vi "ODMR Velmex sweep ACCES DAC control.vi"() -> ()   [LabVIEW 2012]
uses:
  <vilib>/DAQmx/read.llb/DAQmx Read (Counter 1D DBL 1Chan NSamp).vi
  <vilib>/Analysis/1siggen.llb/Ramp Pattern by Samples.vi
  VELMEX step motor/GMW Motion Control_VELMEX_V2_2.llb/Config.vi
  <vilib>/DAQmx/create/channels.llb/DAQmx Create Channel (CI-Count Edges).vi
  <vilib>/DAQmx/configure/timing.llb/DAQmx Timing (Sample Clock).vi
  <vilib>/Utility/file.llb/Write To Spreadsheet File (DBL).vi
  <vilib>/DAQmx/miscellaneous.llb/DAQmx Fill In Error Info.vi
  <resource>/objmgr/daqmx.rc
  <vilib>/Analysis/NI_AALBase.lvlib
panel:
  in  "Home?":bool
  in  "Home T":dbl=50.0
  in  "Home Z":dbl=50.0
  in  "Home Y":dbl=50.0
  in  "Home X":dbl=50.0
  in  "angle":dbl
  in  "angled?":bool
  out "position":dbl
  in  "start":dbl format="%0.2f"
  in  "end":dbl=1.0 format="%0.2f"
  in  "samples":i32=128
  in  "axis":string="T"
  in  "GPIB Address":refnum<visa-resource-name>="GPIB0::1::INSTR"
  in  "datalog path (use dialog)":path
  out "XY Graph":cluster{"Y":dbl[], "Y":dbl[]}[](graph)
  in  "file path (dialog if empty)":path=path "C:/Users/Ouyang Group/Documents/Data/5-13-15/ND Au 686 ODMR sweep 1"
  in  "Z Pos":dbl=52.78
  in  "Y Pos":dbl=112.0
  in  "X Pos":dbl=97.0
  in  "Y Parameters":T1={"Number of Y Steps"=200, "Max Y (V)"=2.0, "Min Y (V)"=-2.0}
  in  "X Parameters":T2={"Number of X Steps"=200, "Max X (V)"=2.0, "Min X (V)"=-2.0}
  in  "RS232 settings":cluster{"Portnumber":i32, "Baudrate":u16}={"Portnumber"=6, "Baudrate"=5} {"Portnumber" items=["COM1", "COM2", "COM3", "COM4", "COM5", "COM6", "COM7", "COM8", "COM9", "COM10", "COM11", "COM12", "COM13", "COM14", "COM15", "COM16", "COM17", "COM18", "COM19", "COM20", "COM21", "COM22", "COM23", "COM24", "COM25", "COM26", "COM27", "COM28", "COM29", "COM30"]; "Baudrate" items=["9600", "14400", "19200", "38400", "57600", "115200"]}
  in  "samples per channel":i32=500
  in  "rate":dbl=100.0 format="%0.2f"
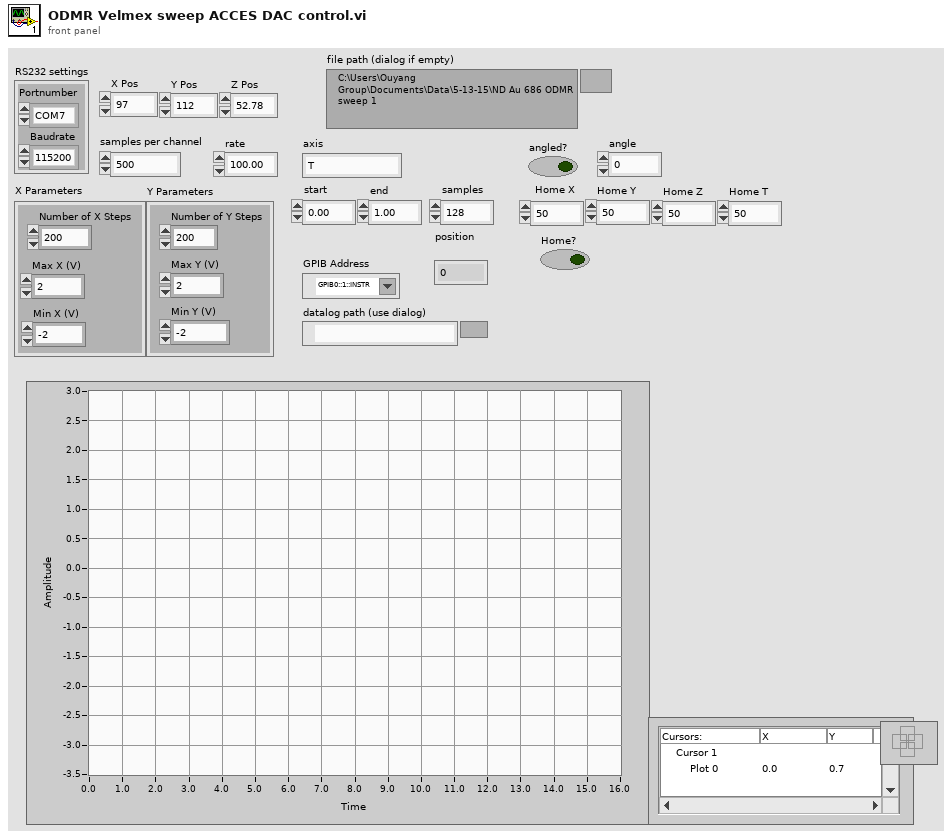
[diagram p1: front panel]
types:
  T1 = cluster{"Number of Y Steps":i32, "Max Y (V)":dbl, "Min Y (V)":dbl}
  T2 = cluster{"Number of X Steps":i32, "Max X (V)":dbl, "Min X (V)":dbl}
  T3 = cluster{"Controller Setup":cluster{"T":string, "Z":string, "Y":string, "X":string, "CW Offset":dbl, "CCW Offset":dbl, "Z Offset":dbl, "Y Offset":dbl, "X Offset":dbl, "Rotary Resolution":i32, "Linear Resolution":i32, "T Speed":dbl, "Z Speed":dbl, "Y Speed":dbl, "X Speed":dbl}, "SoftLimit":cluster{"X soft limit":cluster{"X up soft limit":dbl, "X low soft limit":dbl}, "Y soft limit":cluster{"Y up soft limit":dbl, "Y low soft limit":dbl}, "Z soft limit":cluster{"Z up soft limit":dbl, "Z low soft limit":dbl}, "T soft limit":cluster{"T up soft limit":dbl, "T low soft limit":dbl}}}
  T4 = cluster{"T":string, "Z":string, "Y":string, "X":string, "CW Offset":dbl, "CCW Offset":dbl, "Z Offset":dbl, "Y Offset":dbl, "X Offset":dbl, "Rotary Resolution":i32, "Linear Resolution":i32, "T Speed":dbl, "Z Speed":dbl, "Y Speed":dbl, "X Speed":dbl}
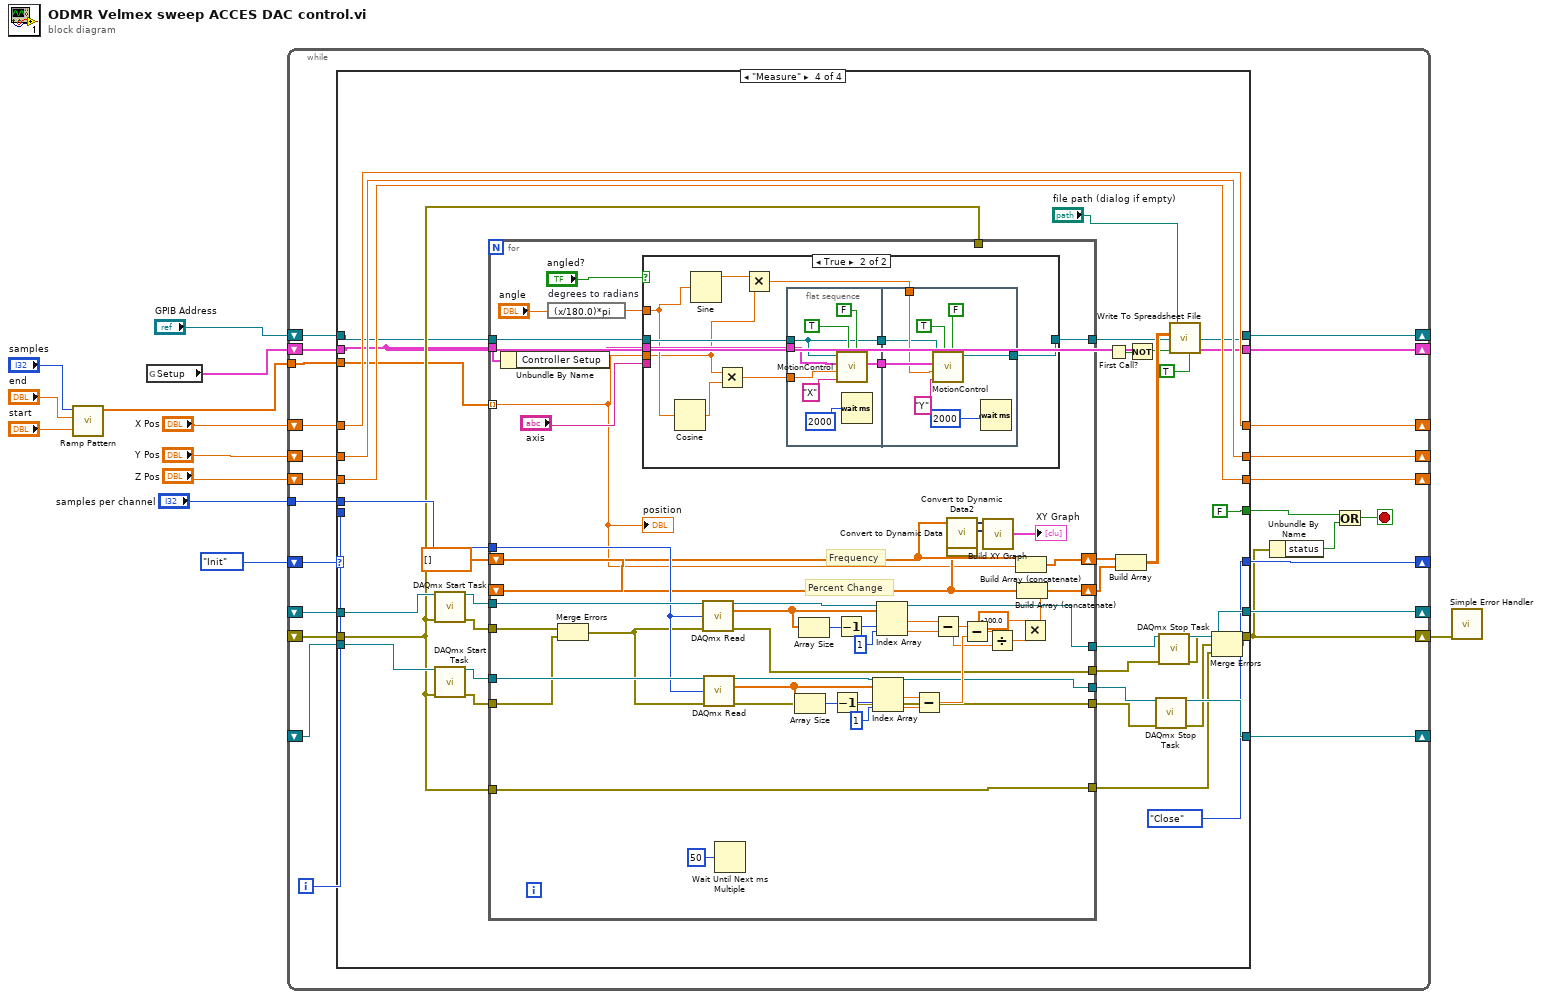
[diagram p0: block diagram]
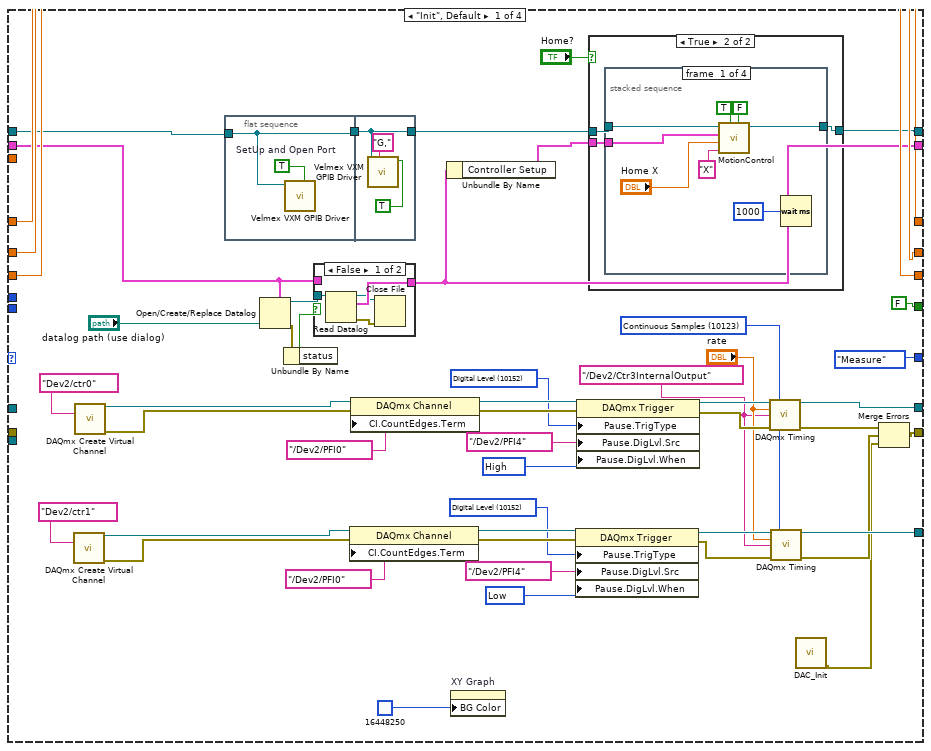
[diagram p2: hidden frame]
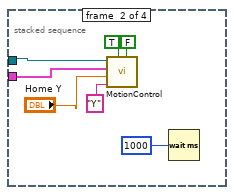
[diagram p4: hidden frame]
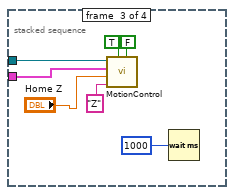
[diagram p5: hidden frame]
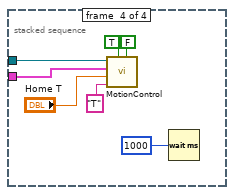
[diagram p6: hidden frame]
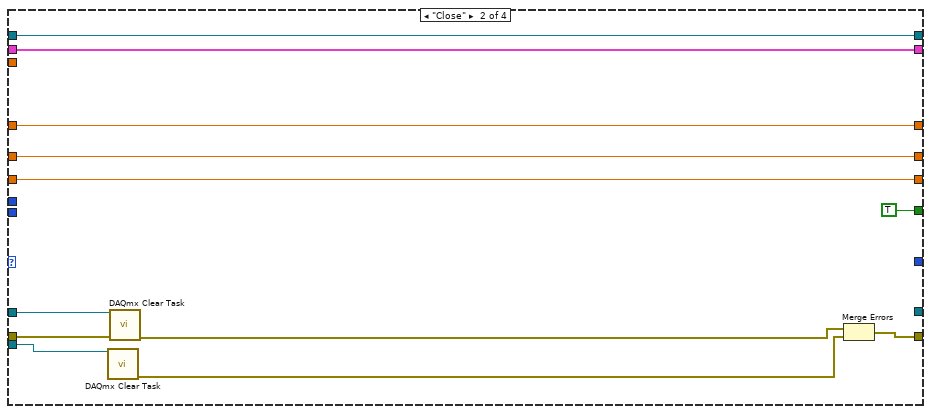
[diagram p8: hidden frame]
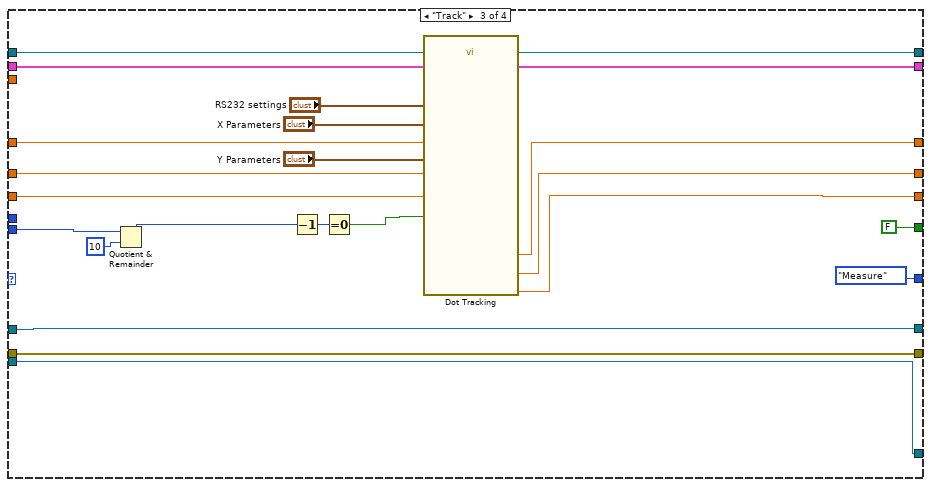
[diagram p9: hidden frame]
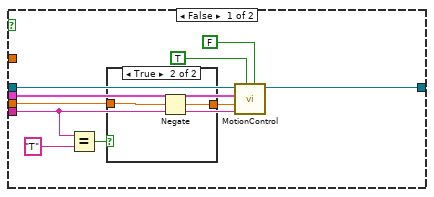
[diagram p10: hidden frame]
diagram:
  n1 = call-poly <vilib>:"Ramp Pattern.vi"("start"="start", "end"="end", "samples"="samples") -> ("Ramp Pattern"=w1:dbl[])  [unwired: 7 in, 1 out]
  n2 = global read "Config.vi" "Setup"() -> (w5:T3)
  n3 = while {
    shift-right: [w33] -> _
    shift-left: enum16{"Init", "Measure", "Track", "Close"}."Init" -> [w36]
    shift-right: [w35] -> _
    shift-left: _ -> [w32]
    shift-right: [w34] -> _
    shift-left: _ -> [w31]
    shift-right: [w28] -> w10
    shift-left: _ -> [w30]
    tunnel: "samples per channel" -> [w25]
    shift-right: [w20] -> _
    shift-left: "X Pos" -> [w23]
    shift-right: [w19] -> _
    shift-left: "Y Pos" -> [w22]
    shift-right: [w18] -> _
    shift-left: "Z Pos" -> [w21]
    shift-right: [w17] -> _
    shift-left: "GPIB Address" -> [w14]
    shift-right: [w16] -> _
    shift-left: w5 -> [w15]
    tunnel: w1 -> [w13]
    i -> [w29]
    stop <- w27 stop-if-true
    n4 = case shown="\"Measure\"" w36 {
      tunnel: [FALSE TRUE FALSE FALSE] -> w26
      tunnel: [w60 _ w161 w186] -> w35
      tunnel: [w59 _ w160 w183] -> w34
      tunnel: [w56 w135 w151 w196] -> w28
      tunnel: [enum16{"Init", "Measure", "Track", "Close"}."Measure" _ enum16{"Init", "Measure", "Track", "Close"}."Measure" enum16{"Init", "Measure", "Track", "Close"}."Close"] -> w33
      tunnel: w32 -> [_ w139 w161 w192]
      tunnel: w31 -> [_ w137 w160 w189]
      tunnel: w30 -> [_ w138 w151 w168]
      tunnel: w29 -> [_ _ w152 _]
      tunnel: w25 -> [_ _ _ w174]
      tunnel: w23 -> [w52 w133 w148 w172]
      tunnel: w22 -> [w51 w132 w147 w171]
      tunnel: w21 -> [w50 w131 w146 w170]
      tunnel: [w52 w133 w145 w172] -> w20
      tunnel: [w51 w132 w144 w171] -> w19
      tunnel: [w50 w131 w143 w170] -> w18
      tunnel: [w40 w130 w142 w163] -> w17
      tunnel: [w39 w129 w141 w164] -> w16
      tunnel: w14 -> [w43 w130 w142 w165]
      tunnel: w15 -> [w42 w129 w141 w164]
      tunnel: w13 -> [_ _ _ w162]
      frame "Init", Default {
        w61 = tag "/Dev2/Ctr3InternalOutput" ("source")
        w63 = 10123 items=["Finite Samples"=10178, "Continuous Samples"=10123, "Hardware Timed Single Point"=12522] ("sample mode")
        w68 = 10214 items=["High"=10192, "Low"=10214] ("Pause.DigLvl.When")
        w70 = 10152 items=["Analog Level"=10101, "Analog Window"=10103, "Digital Level"=10152, "Digital Pattern"=10398, "None"=10230] ("Pause.TrigType")
        w77 = 10192 items=["High"=10192, "Low"=10214] ("Pause.DigLvl.When")
        w79 = 10152 items=["Analog Level"=10101, "Analog Window"=10103, "Digital Level"=10152, "Digital Pattern"=10398, "None"=10230] ("Pause.TrigType")
        n5 = call-poly <vilib>:"DAQmx Create Virtual Channel.vi"("counter"=tag "Dev2/ctr1") -> ("task out"=w75:refnum<k21>, "error out"=w74:errorcluster)  [unwired: 13 in]
        n6 = call-poly <vilib>:"DAQmx Create Virtual Channel.vi"("counter"=tag "Dev2/ctr0") -> ("task out"=w84:refnum<k21>, "error out"=w83:errorcluster)  [unwired: 13 in]
        n7 = flat-sequence {
          tunnel: w43 -> [w119]
          tunnel: [w119] -> w48
          tunnel: [w123] -> w41
          tunnel: w48 -> [w123]
          frame #0 {
            w120 = TRUE  # SetUp and Open Port
            n8 = call "Velmex VXM GPIB Driver.vi"("SetUp and Open Port"=w120, "VISA resource name"=w119) -> ()  [unwired: 8 in, 2 out]
          }
          frame #1 {
            n9 = call "Velmex VXM GPIB Driver.vi"("Send String to VXM"=TRUE, "String to send to VXM"="G,", "VISA resource name"=w123) -> ()  [unwired: 7 in, 2 out]
          }
        }
        n10 = Open/Create/Replace Datalog(5:w42, 11:"datalog path (use dialog)") -> (0:w47:errorcluster, 3:w46:refnum<k1>)  [unwired: 4 in, 1 out]
        n11 = Unbundle By Name(w47) -> ("status"=w45:bool)
        n12 = case shown="False" w45 {
          tunnel: w46 -> [w124 _]
          tunnel: [w127 w128] -> w39
          tunnel: w42 -> [_ w128]
          frame False {
            n13 = Read Datalog(7:w124) -> (0:w126:errorcluster, 2:w127:T3, 3:w125:refnum<k1>)  [unwired: 2 in]
            n14 = Close File(refnum=w125, error in=w126) -> ()  [unwired: 2 out]
          }
          frame True {
          }
        }
        n15 = property class="DAQmx Channel"(reference=w75, error in=w74, "CI.CountEdges.Term"=tag "/Dev2/PFI0") -> (reference out=w72:refnum<k21>, error out=w71:errorcluster)
        n16 = property class="DAQmx Channel"(reference=w84, error in=w83, "CI.CountEdges.Term"=tag "/Dev2/PFI0") -> (reference out=w81:refnum<k21>, error out=w80:errorcluster)
        n17 = Unbundle By Name(w39) -> ("Controller Setup"=w38:T4)
        n18 = property on="XY Graph" class="XYGraph (strict)"("BG Color"=u32 16448250) -> ()  [unwired: 2 in, 2 out]
        n19 = property class="DAQmx Trigger"(reference=w72, error in=w71, "Pause.TrigType"=w70, "Pause.DigLvl.Src"=tag "/Dev2/PFI4", "Pause.DigLvl.When"=w68) -> (reference out=w65:refnum<k21>, error out=w64:errorcluster)
        n20 = property class="DAQmx Trigger"(reference=w81, error in=w80, "Pause.TrigType"=w79, "Pause.DigLvl.Src"=tag "/Dev2/PFI4", "Pause.DigLvl.When"=w77) -> (reference out=w67:refnum<k21>, error out=w66:errorcluster)
        n21 = case shown="True" "Home?" {
          tunnel: w41 -> [w86 w89]
          tunnel: [w86 w88] -> w40
          tunnel: w38 -> [_ w87]
          frame False {
          }
          frame True {
            n22 = stacked-sequence {
              tunnel: [w91 _ _ _] -> w88
              tunnel: w87 -> [w92 w99 w109 w113]
              tunnel: w89 -> [w93 w100 w110 w114]
              frame #0 {
                n23 = call "MotionControl.vi"("STOP motion"=FALSE, "START motion"=TRUE, "axis"="X", "Position"="Home X", "Setup"=w92, "VISA resource name in"=w93) -> ("VISA resource name out"=w91:refnum<visa-resource-name>)  [unwired: 3 in]
                n24 = Wait (ms)(milliseconds to wait=u32 1000) -> ()  [unwired: 1 out]
              }
              frame #1 {
                n25 = call "MotionControl.vi"("STOP motion"=FALSE, "START motion"=TRUE, "axis"="Y", "Position"="Home Y", "Setup"=w99, "VISA resource name in"=w100) -> ()  [unwired: 3 in, 1 out]
                n26 = Wait (ms)(milliseconds to wait=u32 1000) -> ()  [unwired: 1 out]
              }
              frame #2 {
                n27 = call "MotionControl.vi"("STOP motion"=FALSE, "START motion"=TRUE, "axis"="Z", "Position"="Home Z", "Setup"=w109, "VISA resource name in"=w110) -> ()  [unwired: 3 in, 1 out]
                n28 = Wait (ms)(milliseconds to wait=u32 1000) -> ()  [unwired: 1 out]
              }
              frame #3 {
                n29 = call "MotionControl.vi"("STOP motion"=FALSE, "START motion"=TRUE, "axis"="T", "Position"="Home T", "Setup"=w113, "VISA resource name in"=w114) -> ()  [unwired: 3 in, 1 out]
                n30 = Wait (ms)(milliseconds to wait=u32 1000) -> ()  [unwired: 1 out]
              }
            }
          }
        }
        n31 = call-poly <vilib>:"DAQmx Timing.vi"("task/channels in"=w67, "sample mode"=w63, "rate"="rate", "source"=w61, "error in"=w66) -> ("task out"=w60:refnum<k21>, "error out"=w58:errorcluster)  [unwired: 9 in]
        n32 = call-poly <vilib>:"DAQmx Timing.vi"("task/channels in"=w65, "sample mode"=w63, "rate"="rate", "source"=w61, "error in"=w64) -> ("task out"=w59:refnum<k21>, "error out"=w57:errorcluster)  [unwired: 9 in]
        n33 = call "DAC_Init.vi"() -> ("error out"=w49:errorcluster)  [unwired: 11 in]
        n34 = Merge Errors(w58, w57, w49) -> (w56:errorcluster)
      }
      frame "Close" {
        n35 = call <vilib>:"DAQmx Clear Task.vi"("task in"=w137) -> ("error out"=w136:errorcluster)  [unwired: 14 in]
        n36 = call <vilib>:"DAQmx Clear Task.vi"("task in"=w139, "error in"=w138) -> ("error out"=w134:errorcluster)  [unwired: 13 in]
        n37 = Merge Errors(w134, w136) -> (w135:errorcluster)
      }
      frame "Track" {
        n38 = Quotient & Remainder(x=w152, y=10) -> (x-y*floor(x/y)=w155:i32)  [unwired: 1 out]
        n39 = Decrement(x=w155) -> (x-1=w156:i32)
        n40 = Equal To 0?(x=w156) -> (x = 0?=w153:bool)
        n41 = call "Dot Tracking.vi"("X"="X Parameters", "Y Parameters"="Y Parameters", "RS232 settings"="RS232 settings", "X Pos"=w148, "Y pos"=w147, "Z Pos"=w146, "Z-track?"=w153) -> ("X Position"=w145:dbl, "Y Position"=w144:dbl, "Z Position"=w143:dbl)  [unwired: 2 in, 4 out]
      }
      frame "Measure" {
        w173 = dbl[] []
        n42 = call <vilib>:"DAQmx Start Task.vi"("task/channels in"=w192, "error in"=w168) -> ("task out"=w190:refnum<k21>, "error out"=w191:errorcluster)  [unwired: 12 in]
        n43 = call <vilib>:"DAQmx Start Task.vi"("task/channels in"=w189, "error in"=w168) -> ("task out"=w188:refnum<k21>, "error out"=w187:errorcluster)  [unwired: 12 in]
        n44 = for {
          shift-right: [w229] -> w180
          shift-left: w173 -> [w215]
          shift-right: [w228] -> w181
          shift-left: w173 -> [w217]
          tunnel: w188 -> [w224]
          tunnel: [w223] -> w185
          tunnel: [w222] -> w194
          tunnel: [w219] -> w193
          tunnel: w191 -> [w221]
          tunnel: w190 -> [w220]
          tunnel: w187 -> [w210]
          tunnel: w174 -> [w218]
          tunnel: w168 -> [_]
          tunnel: [w208] -> w169
          tunnel: w168 -> [w201]
          tunnel: [w201] -> w167
          tunnel: w165 -> [w206]
          tunnel: w164 -> [w205]
          tunnel: [w202] -> w163
          tunnel: w162 -> [w200] mode=indexing
          # "Percent Change"
          # "Frequency"
          n45 = Unbundle By Name(w205) -> ("Controller Setup"=w203:T4)
          n46 = expression code="(x/180.0)*pi" "degrees to radians"("angle") -> (w197:dbl)
          n47 = Merge Errors(w221, w210) -> (w209:errorcluster)
          n48 = case shown="True" "angled?" {
            tunnel: w206 -> [w250 w266]
            tunnel: "axis" -> [w247 _]
            tunnel: w203 -> [w249 w265]
            tunnel: [w248 w260] -> w202
            tunnel: w200 -> [w244 w258]
            tunnel: w197 -> [_ w264]
            frame False {
              n49 = Equal?(x=w247, y="T") -> (x = y?=w245:bool)
              n50 = case shown="True" w245 {
                tunnel: w244 -> [w253 w255]
                tunnel: [w253 w254] -> w243
                frame False {
                }
                frame True {
                  n51 = Negate(x=w255) -> (-x=w254:dbl)
                }
              }
              n52 = call "MotionControl.vi"("STOP motion"=FALSE, "START motion"=TRUE, "axis"=w247, "Position"=w243, "Setup"=w249, "VISA resource name in"=w250) -> ("VISA resource name out"=w248:refnum<visa-resource-name>)  [unwired: 3 in]
            }
            frame True {
              n53 = Cosine(x=w264) -> (cos(x)=w263:dbl)
              n54 = Sine(x=w264) -> (sin(x)=w259:dbl)
              n55 = Multiply(x=w258, y=w263) -> (x*y=w262:dbl)
              n56 = Multiply(x=w259, y=w258) -> (x*y=w257:dbl)
              n57 = flat-sequence {
                tunnel: w266 -> [w268]
                tunnel: w265 -> [w267]
                tunnel: w262 -> [w270]
                tunnel: [w267] -> w261
                tunnel: [w268] -> w256
                tunnel: w261 -> [w278]
                tunnel: [w277] -> w260
                tunnel: w257 -> [w276]
                tunnel: w256 -> [w275]
                frame #0 {
                  n58 = call "MotionControl.vi"("STOP motion"=FALSE, "START motion"=TRUE, "axis"="X", "Position"=w270, "Setup"=w267, "VISA resource name in"=w268) -> ()  [unwired: 3 in, 1 out]
                  n59 = Wait (ms)(milliseconds to wait=u32 2000 ("millisecond multiple")) -> ()  [unwired: 1 out]
                }
                frame #1 {
                  n60 = call "MotionControl.vi"("STOP motion"=FALSE, "START motion"=TRUE, "axis"="Y", "Position"=w276, "Setup"=w278, "VISA resource name in"=w275) -> ("VISA resource name out"=w277:refnum<visa-resource-name>)  [unwired: 3 in]
                  n61 = Wait (ms)(milliseconds to wait=u32 2000 ("millisecond multiple")) -> ()  [unwired: 1 out]
                }
              }
            }
          }
          n62 = call-poly <vilib>:"DAQmx Read.vi"("task/channels in"=w220, "number of samples per channel"=w218, "error in"=w209) -> ("task out"=w222:refnum<k21>, "data"=w242:dbl[], "error out"=w223:errorcluster)  [unwired: 10 in]
          n63 = call-poly <vilib>:"DAQmx Read.vi"("task/channels in"=w224, "number of samples per channel"=w218, "error in"=w209) -> ("task out"=w219:refnum<k21>, "data"=w231:dbl[], "error out"=w208:errorcluster)  [unwired: 10 in]
          n64 = Wait Until Next ms Multiple(millisecond multiple=u32 50) -> ()  [unwired: 1 out]
          n65 = Array Size(array=w231) -> (size(s)=w236:i32)
          n66 = Array Size(array=w242) -> (size(s)=w241:i32)
          n67 = Decrement(x=w236) -> (x-1=w235:i32)
          n68 = Decrement(x=w241) -> (x-1=w240:i32)
          n69 = Index Array(array=w231, index #1=w235, index #2=1 ("index")) -> (element #1=w232:dbl, element #2=w233:dbl)
          n70 = Index Array(array=w242, index #1=w240, index #2=1 ("index")) -> (element #1=w237:dbl, element #2=w238:dbl)
          n71 = Subtract(x=w232, y=w233) -> (x-y=w230:dbl)
          n72 = Subtract(x=w237, y=w238) -> (x-y=w226:dbl)
          n73 = call "Convert to Dynamic Data"("Array"=w217) -> ("Dynamic Data Type"=w216:dynamicdata)  [unwired: 3 in]
          n74 = call "Convert to Dynamic Data2"("Array"=w215) -> ("Dynamic Data Type"=w214:dynamicdata)  [unwired: 3 in]
          n75 = Subtract(x=w226, y=w230) -> (x-y=w227:dbl)
          n76 = call "Build XY Graph"("Y Input"=w214, "X Input"=w216) -> ("XY Graph"=→"XY Graph":cluster{"Y":dbl[], "Y":dbl[]}[])  [unwired: 3 in, 6 out]
          n77 = Divide(x=w227, y=w226) -> (x/y=w225:dbl)
          n78 = Build Array (concatenate)(w217, w200) -> (w228:dbl[])
          n79 = Multiply(x=-100.0, y=w225) -> (x*y=w212:dbl)
          n80 = Build Array (concatenate)(w215, w212) -> (w229:dbl[])
          "position" <- w200
        }
        n81 = First Call?() -> (First Call?: T/F=w178:bool)
        n82 = Build Array(w181, w180) -> (w179:dbl[][])
        n83 = Not(x=w178) -> (.not. x?=w177:bool)
        n84 = call <vilib>:"DAQmx Stop Task.vi"("task/channels in"=w193, "error in"=w169) -> ("task out"=w183:refnum<k21>, "error out"=w182:errorcluster)  [unwired: 12 in]
        n85 = call <vilib>:"DAQmx Stop Task.vi"("task/channels in"=w194, "error in"=w185) -> ("task out"=w186:refnum<k21>, "error out"=w184:errorcluster)  [unwired: 12 in]
        n86 = call-poly <vilib>:"Write To Spreadsheet File.vi"("transpose? (no:F)"=TRUE, "append to file? (new file:F)"=w177, "2D data"=w179, "file path (dialog if empty)"="file path (dialog if empty)") -> ()  [unwired: 4 in, 1 out]
        n87 = Merge Errors(w184, w182, w167) -> (w196:errorcluster)
      }
    }
    n88 = Unbundle By Name(w28) -> ("status"=w24:bool)
    n89 = Or(x=w26, y=w24) -> (x .or. y?=w27:bool)
  }
  n90 = call <vilib>:"Simple Error Handler.vi"("error in (no error)"=w10) -> ()  [unwired: 4 in, 5 out]
